vi "2013_01_03 Durability8 Main.vi"() -> ()   [LabVIEW 2011]
uses:
  <vilib>/DAQmx/write.llb/DAQmx Write (Counter Time 1Chan 1Samp).vi
  <vilib>/measure/NI_MAPro.lvlib
  <vilib>/measure/madcrms.llb/Averaged DC-RMS for N Chan.vi
  <vilib>/DAQmx/read.llb/DAQmx Read (Analog 1D Wfm NChan NSamp).vi
  <vilib>/Utility/TradDaqScaling.llb/Convert Thermistor Reading (waveform).vi
  MotorTypeDef.ctl
panel:
  out "Saving Data 2":bool caption="Saving Data"
  in  "new_file event":bool caption="new_file"
  out "Saving Data":bool
  in  "File Path":path=path "Durability/fine.lvm"
  out "Voltages":waveform(dbl)[](graph)
  out "Currents":waveform(dbl)[](graph)
  in  "Motor 8":T1 {"Elapsed Time" format="%<%H:%M:%S>t"; "Efficiency" format="%#_3g%%"; "Supply Voltage (V)" format="%#_3f"; "Power Output (W)" format="%#_3g"; "Power Usage (W)" format="%#_3g"; "Torque (mNm)" format="%#_3g"; "RPM" scale=0.0..40000.0 scale format="%#.6p"}
  in  "Motor 7":T1 {"Elapsed Time" format="%<%H:%M:%S>t"; "Efficiency" format="%#_3g%%"; "Supply Voltage (V)" format="%#_3f"; "Power Output (W)" format="%#_3g"; "Power Usage (W)" format="%#_3g"; "Torque (mNm)" format="%#_3g"; "RPM" scale=0.0..40000.0 scale format="%#.6p"}
  in  "Motor 6":T1 {"Elapsed Time" format="%<%H:%M:%S>t"; "Efficiency" format="%#_3g%%"; "Supply Voltage (V)" format="%#_3f"; "Power Output (W)" format="%#_3g"; "Power Usage (W)" format="%#_3g"; "Torque (mNm)" format="%#_3g"; "RPM" scale=0.0..40000.0 scale format="%#.6p"}
  in  "Motor 5":T1 {"Elapsed Time" format="%<%H:%M:%S>t"; "Efficiency" format="%#_3g%%"; "Supply Voltage (V)" format="%#_3f"; "Power Output (W)" format="%#_3g"; "Power Usage (W)" format="%#_3g"; "Torque (mNm)" format="%#_3g"; "RPM" scale=0.0..40000.0 scale format="%#.6p"}
  in  "Motor 4":T1 {"Elapsed Time" format="%<%H:%M:%S>t"; "Efficiency" format="%#_3g%%"; "Supply Voltage (V)" format="%#_3f"; "Power Output (W)" format="%#_3g"; "Power Usage (W)" format="%#_3g"; "Torque (mNm)" format="%#_3g"; "RPM" scale=0.0..40000.0 scale format="%#.6p"}
  in  "Motor 3":T1 {"Elapsed Time" format="%<%H:%M:%S>t"; "Efficiency" format="%#_3g%%"; "Supply Voltage (V)" format="%#_3f"; "Power Output (W)" format="%#_3g"; "Power Usage (W)" format="%#_3g"; "Torque (mNm)" format="%#_3g"; "RPM" scale=0.0..40000.0 scale format="%#.6p"}
  in  "Motor 2":T1 {"Elapsed Time" format="%<%H:%M:%S>t"; "Efficiency" format="%#_3g%%"; "Supply Voltage (V)" format="%#_3f"; "Power Output (W)" format="%#_3g"; "Power Usage (W)" format="%#_3g"; "Torque (mNm)" format="%#_3g"; "RPM" scale=0.0..40000.0 scale format="%#.6p"}
  in  "Motor 1":T1 {"Elapsed Time" format="%<%H:%M:%S>t"; "Efficiency" format="%#_3g%%"; "Supply Voltage (V)" format="%#_3f"; "Power Output (W)" format="%#_3g"; "Power Usage (W)" format="%#_3g"; "Torque (mNm)" format="%#_3g"; "RPM" scale=0.0..40000.0 scale format="%#.6p"}
  out "Motor Temp":dbl(slide) scale=90.0..110.0
  out "Tank Temp":dbl(slide) scale=90.0..110.0
  out "RMS Voltages":waveform(dbl)[](graph)
  out "RMS Currents":waveform(dbl)[](graph)
  in  "Temp Probe\nOn Motor":dbl=1.0
  out "loop time (ms)":u32
  in  "stop":bool
  in  "Unlock PWM":bool=TRUE
  in  "PWM 2":dbl(slide)=100.0 min=0.0 max=100.0 step=5.0 scale=0.0..100.0
  in  "PWM 1":dbl(slide) min=0.0 max=100.0 step=5.0 scale=0.0..100.0
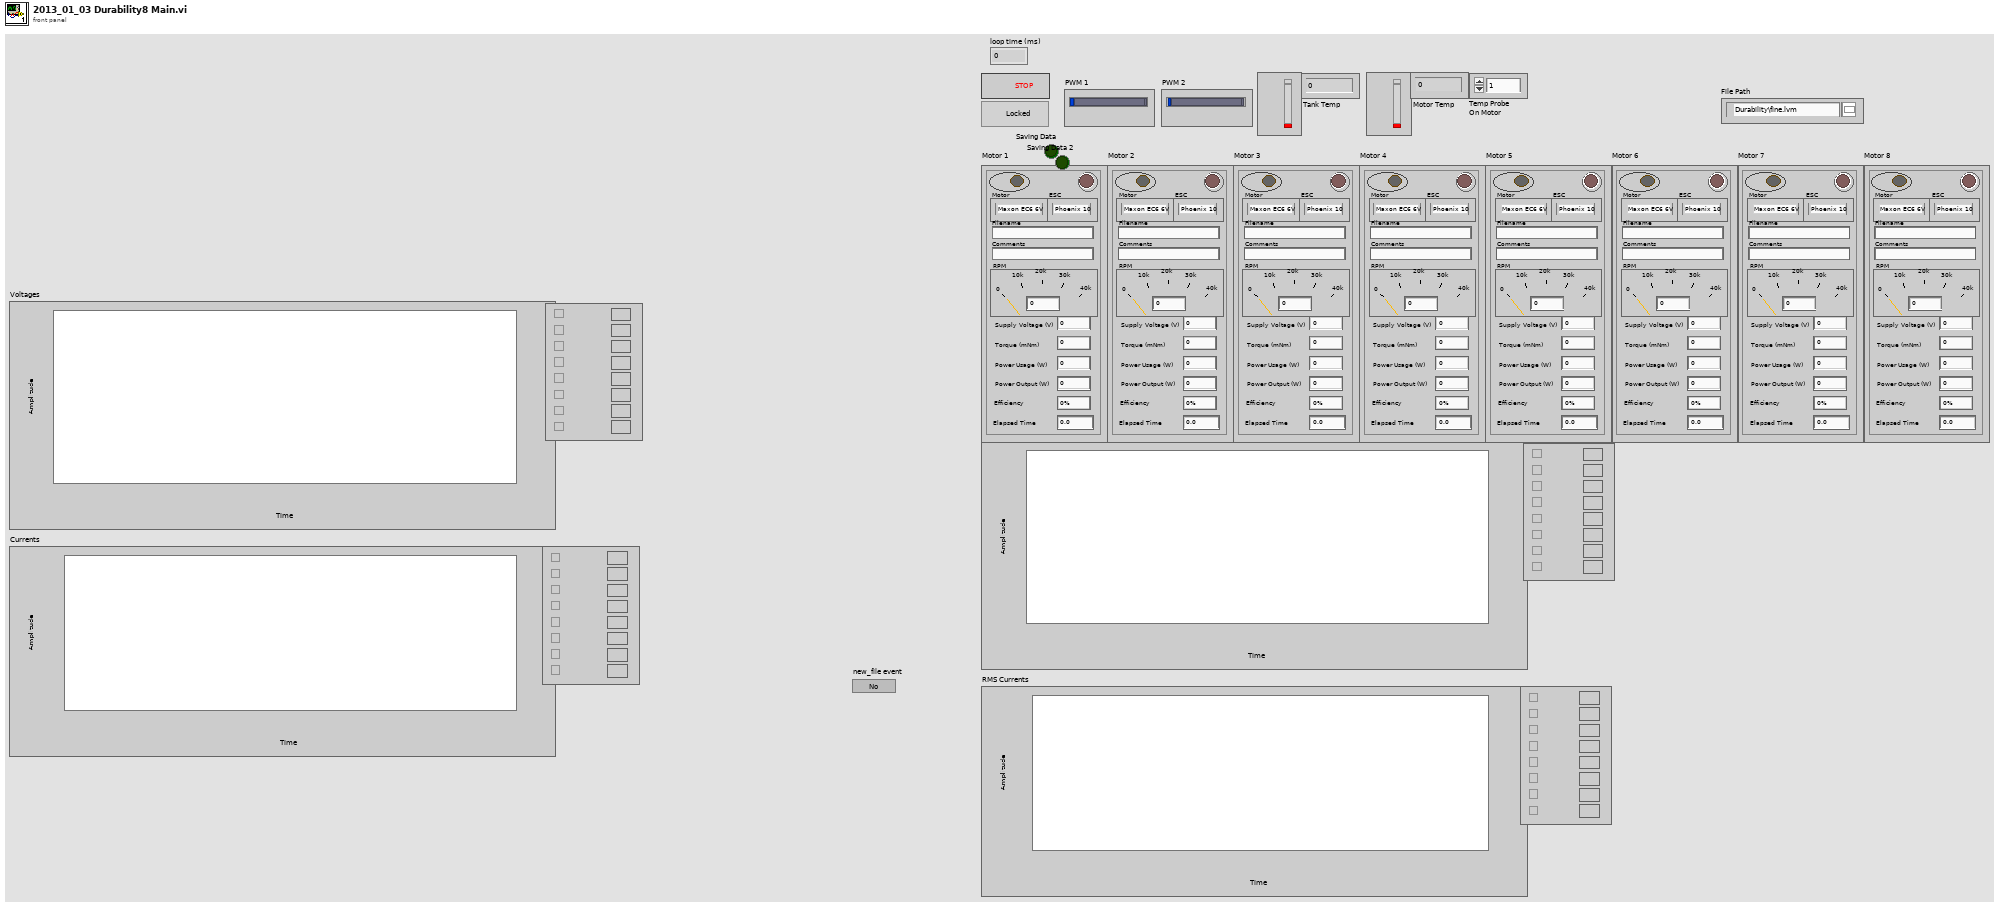
[diagram p1: front panel]
types:
  T1 = typedef "MotorTypeDef.ctl" = cluster{"Enabled":bool, "Fail":bool, "RPM":dbl, "Motor":enum16{"Maxon EC6 6V", "Maxon EC4 6V", "FH 0620 6V", "FH 0620 12V"}, "ESC":enum16{"Phoenix 10", "Maxon", "FH 1801"}, "Torque (mNm)":dbl, "Power Usage (W)":dbl, "Power Output (W)":dbl, "Supply Voltage (V)":dbl, "Efficiency":dbl, "Filename":string, "Comments":string, "Elapsed Time":dbl}
  T2 = enum8{"Enabled", "Disabled", "Disabled and Grayed Out"}
  T3 = enum16{"open", "open or create", "create or replace", "create", "open (read-only)"}
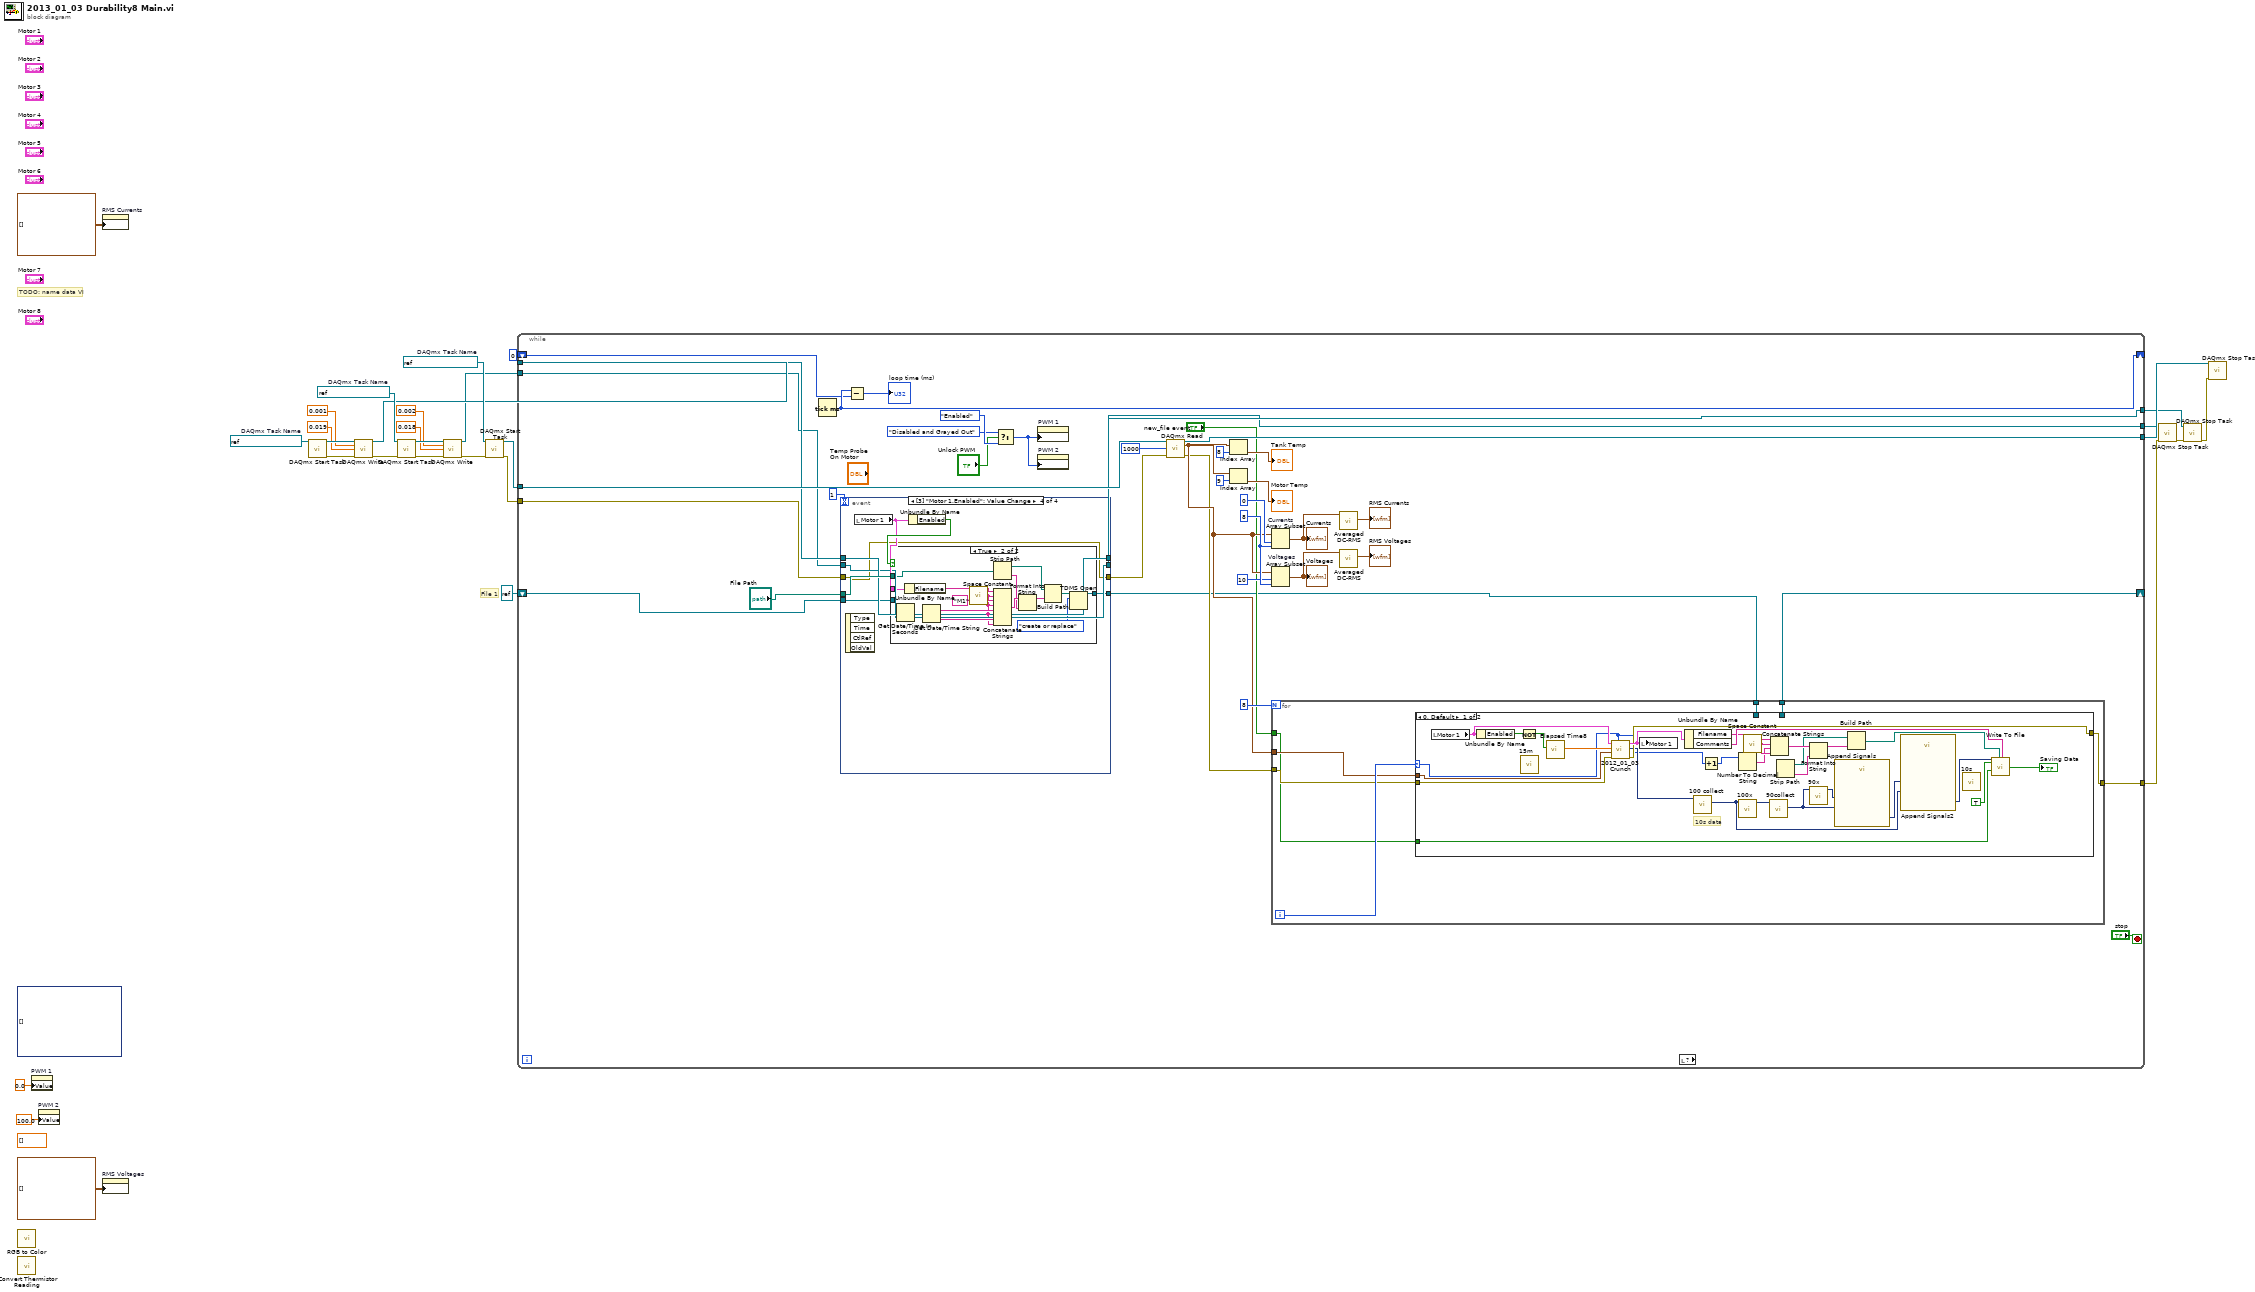
[diagram p0: block diagram]
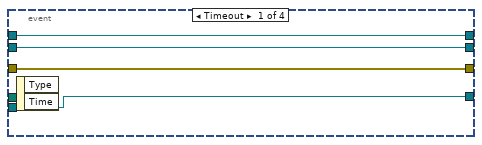
[diagram p2: hidden frame]
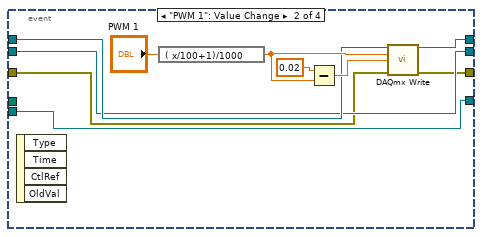
[diagram p3: hidden frame]
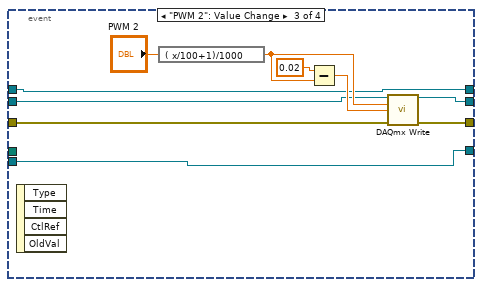
[diagram p4: hidden frame]
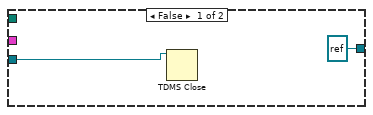
[diagram p5: hidden frame]
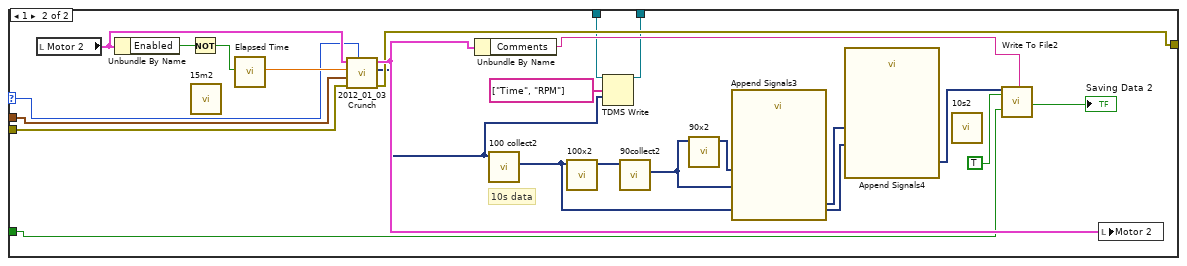
[diagram p6: hidden frame]
diagram:
  (unwired) dynamicdata[] []
  (unwired) dbl[] [] ("History Data")
  w24 = refnum<k21> "Durability8 PWM2"  # DAQmx Task Name
  w25 = refnum<k21> "Durability8 PWM1"  # DAQmx Task Name
  w29 = refnum<k21> "Durability8 Acquire"  # DAQmx Task Name
  # "File 1"
  # "TODO: name data VI"
  n1 = call <vilib>:"RGB to Color.vi"() -> ()  [unwired: 3 in, 1 out]
  n2 = call-poly <vilib>:"Convert Thermistor Reading.vi"() -> ()  [unwired: 7 in, 1 out]
  n3 = property on="PWM 1" class="Slide (strict)"("Value"=0.0 ("PWM 1")) -> ()  [unwired: 2 in, 2 out]
  n4 = property on="PWM 2" class="Slide (strict)"("Value"=100.0 ("PWM 2")) -> ()  [unwired: 2 in, 2 out]
  n5 = property on="RMS Currents" class="WFChart (strict)"("History Data"=waveform(dbl)[][] []) -> ()  [unwired: 2 in, 2 out]
  n6 = property on="RMS Voltages" class="WFChart (strict)"("History Data"=waveform(dbl)[][] []) -> ()  [unwired: 2 in, 2 out]
  n7 = call <vilib>:"DAQmx Start Task.vi"("task/channels in"=w25) -> ("task out"=w21:refnum<k21>, "error out"=w19:errorcluster)  [unwired: 13 in]
  n8 = call-poly <vilib>:"DAQmx Write.vi"("task/channels in"=w21, "high time"=0.001 ("data"), "low time"=0.019 ("data"), "error in"=w19) -> ("task out"=w23:refnum<k21>, "error out"=w18:errorcluster)  [unwired: 9 in, 1 out]
  n9 = call <vilib>:"DAQmx Start Task.vi"("task/channels in"=w24, "error in"=w18) -> ("task out"=w20:refnum<k21>, "error out"=w17:errorcluster)  [unwired: 12 in]
  n10 = call-poly <vilib>:"DAQmx Write.vi"("task/channels in"=w20, "high time"=0.002 ("data"), "low time"=0.018 ("data"), "error in"=w17) -> ("task out"=w22:refnum<k21>, "error out"=w16:errorcluster)  [unwired: 9 in, 1 out]
  n11 = call <vilib>:"DAQmx Start Task.vi"("task/channels in"=w29, "error in"=w16) -> ("task out"=w28:refnum<k21>, "error out"=w26:errorcluster)  [unwired: 12 in]
  n12 = while {
    tunnel: w28 -> [w67]
    tunnel: [w66] -> w27
    tunnel: w26 -> [w43]
    shift-right: [w60] -> _
    shift-left: u32 0 ("millisecond timer value") -> [w59]
    tunnel: w23 -> [w45]
    tunnel: w22 -> [w44]
    tunnel: [w42] -> w15
    tunnel: [w41] -> w6
    tunnel: [w34] -> w2
    shift-right: [w30] -> _
    shift-left: refnum<k34> refnum ("tdms file out") -> [w32]
    stop <- "stop" stop-if-true
    w55 = 8 ("length")
    n13 = Tick Count (ms)() -> (millisecond timer value=w60:u32)
    n14 = event shown="[3] \"Motor 1.Enabled\": Value Change" {
      selector: _ -> [_ _ _ _]
      dyn-events: _ -> [_ _ _ _]
      timeout: 1 -> [_ _ _ _]
      tunnel: w45 -> [w71 w77 w84 w96]
      tunnel: w44 -> [w70 w75 w83 w95]
      tunnel: [w71 w76 w84 w96] -> w42
      tunnel: [w70 w75 w85 w95] -> w41
      tunnel: [w69 w74 w86 w94] -> w37
      tunnel: w43 -> [w69 w73 w87 w94]
      tunnel: "File Path" -> [_ _ _ w99]
      tunnel: [w68 w72 w82 w93] -> w31
      tunnel: w32 -> [w68 w72 w82 w92]
      event Timeout {
        n15 = event-data() -> ()  [unwired: 1 in, 2 out]
      }
      event "PWM 1": Value Change {
        n16 = event-data() -> ()  [unwired: 1 in, 4 out]
        n17 = expression code="( x/100+1)/1000"("PWM 1") -> (w78:dbl)
        n18 = Subtract(x=0.02 ("y"), y=w78) -> (x-y=w79:dbl)
        n19 = call-poly <vilib>:"DAQmx Write.vi"("task/channels in"=w77, "high time"=w78, "low time"=w79, "error in"=w73) -> ("task out"=w76:refnum<k21>, "error out"=w74:errorcluster)  [unwired: 9 in, 1 out]
      }
      event "PWM 2": Value Change {
        n20 = event-data() -> ()  [unwired: 1 in, 4 out]
        n21 = expression code="( x/100+1)/1000"("PWM 2") -> (w91:dbl)
        n22 = Subtract(x=0.02, y=w91) -> (x-y=w89:dbl)
        n23 = call-poly <vilib>:"DAQmx Write.vi"("task/channels in"=w83, "high time"=w91, "low time"=w89, "error in"=w87) -> ("task out"=w85:refnum<k21>, "error out"=w86:errorcluster)  [unwired: 9 in, 1 out]
      }
      event Value Change {
        n24 = event-data() -> ()  [unwired: 1 in, 4 out]
        n25 = local read "Motor 1"() -> (w97:T1)
        n26 = Unbundle By Name(w97) -> ("Enabled"=w98:bool)
        n27 = case shown="True" w98 {
          tunnel: w99 -> [_ w109]
          tunnel: w97 -> [_ w115]
          tunnel: [refnum<k34> refnum ("tdms file out") w102] -> w93
          tunnel: w92 -> [w101 _]
          frame False {
            n28 = TDMS Close(11:w101) -> ()  [unwired: 1 in, 2 out]
          }
          frame True {
            n29 = Get Date/Time In Seconds() -> (seconds since 1Jan1904=w107:timestamp)
            n30 = Unbundle By Name(w115) -> ("Filename"=w110:string)
            n31 = Get Date/Time String(seconds (now)=w107) -> (date string=w105:string, time string=w104:string)  [unwired: 2 in]
            n32 = call <vilib>:"Space Constant.vi"() -> ("String"=w103:string)
            n33 = Strip Path(path=w109) -> (stripped path=w112:path, name=w113:string)
            n34 = Concatenate Strings(w110, w103, "M1" ("string"), w103, w105, w103, w104, w103) -> (w114:string)
            n35 = Format Into String(initial string=w114, w113) -> (resulting string=w111:string)  [unwired: 2 in, 1 out]
            n36 = Build Path(base path=w112, name or relative path=w111) -> (appended path=w108:path)
            n37 = TDMS Open(10:T3."create or replace" ("operation (0:open)"), 11:w108) -> (3:w102:refnum<k34>)  [unwired: 4 in, 1 out]
          }
        }
      }
    }
    n38 = Subtract(x=w60, y=w59) -> (x-y=→"loop time (ms)":u32)
    n39 = Select(t=T2."Disabled and Grayed Out" ("Disabled"), s="Unlock PWM", f=T2."Enabled" ("Disabled")) -> (s? t:f=w64:T2)
    n40 = property on="PWM 1" class="Slide (strict)"("DisabledEnum"=w64) -> ()  [unwired: 2 in, 2 out]
    n41 = property on="PWM 2" class="Slide (strict)"("DisabledEnum"=w64) -> ()  [unwired: 2 in, 2 out]
    n42 = call-poly <vilib>:"DAQmx Read.vi"("task/channels in"=w67, "number of samples per channel"=1000, "error in"=w37) -> ("task out"=w66:refnum<k21>, "data"=w47:waveform(dbl)[], "error out"=w36:errorcluster)  [unwired: 10 in]
    n43 = Index Array(array=w47, index=8) -> (element=→"Tank Temp":waveform(dbl))
    n44 = Index Array(array=w47, index=9) -> (element=→"Motor Temp":waveform(dbl))
    n45 = Array Subset "Currents"(array=w47, index=0, length=w55) -> (w39:waveform(dbl)[])
    "Currents" <- w39
    n46 = Array Subset "Voltages"(array=w47, index=10 ("length"), length=w55) -> (w38:waveform(dbl)[])
    "Voltages" <- w38
    n47 = for {
      N: 8 -> [_]
      tunnel: w47 -> [w122]
      tunnel: w36 -> [w121]
      tunnel: "new_file event" -> [w120]
      tunnel: [w119] -> w34
      tunnel: w31 -> [w118]
      tunnel: [w117] -> w30
      i -> [w123]
      n48 = case shown="0, Default" w123 {
        selector: w123 -> [w124 w157]
        tunnel: w122 -> [w129 w160]
        tunnel: w121 -> [w128 w159]
        tunnel: w120 -> [w131 w162]
        tunnel: [w127 w158] -> w119
        tunnel: w118 -> [_ w156]
        tunnel: [_ w155] -> w117
        frame 0, Default {
          # "10s data"
          n49 = local read "Motor 1"() -> (w150:T1)
          n50 = Unbundle By Name(w150) -> ("Enabled"=w152:bool)
          n51 = Not(x=w152) -> (.not. x?=w151:bool)
          n52 = call "15m"() -> ()  [unwired: 12 in, 8 out]
          n53 = call "Elapsed Time8"("Reset"=w151) -> ("Elapsed Time (s)"=w130:dbl)  [unwired: 11 in, 7 out]
          n54 = call "2012_01_03 Crunch.vi"("Numeric Control"=w124, "error in (no error)"=w128, "data"=w129, "Elapsed Time (s)"=w130, "Motor 8"=w150) -> ("error out"=w127:errorcluster, "Dynamic Data Type"=w126:dynamicdata, "Motor 9"=w134:T1)  [unwired: 4 in]
          n55 = local write "Motor 1"(w134) -> ()
          n56 = Unbundle By Name(w134) -> ("Filename"=w132:string, "Comments"=w133:string)
          n57 = call "100 collect"("Signals"=w126) -> ("Collected Signals"=w148:dynamicdata)  [unwired: 9 in, 1 out]
          n58 = Increment(x=w124) -> (x+1=w125:i32)
          n59 = Number To Decimal String(number=w125) -> (decimal integer string=w140:string)  [unwired: 1 in]
          n60 = call "100x"("Signals"=w148) -> ("Mean"=w144:dynamicdata)  [unwired: 8 in, 2 out]
          n61 = call <vilib>:"Space Constant.vi"() -> ("String"=w141:string)
          n62 = call "90collect"("Signals"=w144) -> ("Collected Signals"=w146:dynamicdata)  [unwired: 9 in, 1 out]
          n63 = Concatenate Strings(w132, w141, w140, w141) -> (w142:string)
          n64 = Strip Path() -> (stripped path=w138:path, name=w139:string)  [unwired: 1 in]
          n65 = Format Into String(initial string=w142, w139) -> (resulting string=w137:string)  [unwired: 2 in, 1 out]
          n66 = call "90x"("Signals"=w146) -> ("Mean"=w145:dynamicdata)  [unwired: 8 in, 2 out]
          n67 = call "Append Signals"("Input Signal B"=w146, "Input Signal A"=w145) -> ("Appended Signals"=w147:dynamicdata)  [unwired: 8 in, 1 out]
          n68 = Build Path(base path=w138, name or relative path=w137) -> (appended path=w143:path)
          n69 = call "Append Signals2"("Input Signal B"=w148, "Input Signal A"=w147) -> ("Appended Signals"=w149:dynamicdata)  [unwired: 8 in, 1 out]
          n70 = call "10s"() -> ()  [unwired: 12 in, 8 out]
          n71 = call "Write To File"("Signals"=w149, "Reset"=TRUE, "new_file"=w131, "Filename"=w143, "Comment"=w133) -> ("Saving Data"=→"Saving Data":bool)  [unwired: 12 in, 2 out]
        }
        frame 1 {
          # "10s data"
          n72 = local read "Motor 2"() -> (w173:T1)
          n73 = Unbundle By Name(w173) -> ("Enabled"=w175:bool)
          n74 = Not(x=w175) -> (.not. x?=w174:bool)
          n75 = call "15m2"() -> ()  [unwired: 12 in, 8 out]
          n76 = call "Elapsed Time"("Reset"=w174) -> ("Elapsed Time (s)"=w161:dbl)  [unwired: 11 in, 7 out]
          n77 = call "2012_01_03 Crunch.vi"("Numeric Control"=w157, "error in (no error)"=w159, "data"=w160, "Elapsed Time (s)"=w161, "Motor 8"=w173) -> ("error out"=w158:errorcluster, "Dynamic Data Type"=w153:dynamicdata, "Motor 9"=w164:T1)  [unwired: 4 in]
          n78 = Unbundle By Name(w164) -> ("Comments"=w163:string)
          n79 = call "100 collect2"("Signals"=w153) -> ("Collected Signals"=w171:dynamicdata)  [unwired: 9 in, 1 out]
          n80 = call "100x2"("Signals"=w171) -> ("Mean"=w167:dynamicdata)  [unwired: 8 in, 2 out]
          n81 = TDMS Write(0:w156, 7:string[] ["Time", "RPM"] ("channel name(s) in (Untitled)"), 9:w153) -> (4:w155:refnum<k34>)  [unwired: 3 in, 3 out]
          n82 = call "90collect2"("Signals"=w167) -> ("Collected Signals"=w169:dynamicdata)  [unwired: 9 in, 1 out]
          n83 = call "90x2"("Signals"=w169) -> ("Mean"=w168:dynamicdata)  [unwired: 8 in, 2 out]
          n84 = call "Append Signals3"("Input Signal B"=w169, "Input Signal A"=w168) -> ("Appended Signals"=w170:dynamicdata)  [unwired: 8 in, 1 out]
          n85 = call "Append Signals4"("Input Signal B"=w171, "Input Signal A"=w170) -> ("Appended Signals"=w172:dynamicdata)  [unwired: 8 in, 1 out]
          n86 = call "10s2"() -> ()  [unwired: 12 in, 8 out]
          n87 = call "Write To File2"("Signals"=w172, "Reset"=TRUE, "new_file"=w162, "Comment"=w163) -> ("Saving Data"=→"Saving Data 2":bool)  [unwired: 13 in, 2 out]
          n88 = local write "Motor 2"(w164) -> ()
        }
      }
    }
    n89 = call-poly <vilib>:"Averaged DC-RMS.vi"("signals in"=w39) -> ("RMS value waveforms"=→"RMS Currents":waveform(dbl)[])  [unwired: 6 in, 4 out]
    n90 = call-poly <vilib>:"Averaged DC-RMS.vi"("signals in"=w38) -> ("RMS value waveforms"=→"RMS Voltages":waveform(dbl)[])  [unwired: 6 in, 4 out]
    n91 = local read item#-1() -> ()  [unwired: 1 out]
  }
  n92 = call <vilib>:"DAQmx Stop Task.vi"("task/channels in"=w6, "error in"=w2) -> ("error out"=w14:errorcluster)  [unwired: 12 in, 1 out]
  n93 = call <vilib>:"DAQmx Stop Task.vi"("task/channels in"=w15, "error in"=w14) -> ("error out"=w13:errorcluster)  [unwired: 12 in, 1 out]
  n94 = call <vilib>:"DAQmx Stop Task.vi"("task/channels in"=w27, "error in"=w13) -> ()  [unwired: 12 in, 2 out]
